vi "Get Event Selector Name QD.vi"(8 "error in (no error)":errorcluster, 10 "Library Ref in":refnum<vi>, 11 "VI Ref in":refnum<vi>) -> (0 "error out":errorcluster, 2 "Library Ref out":refnum<vi>, 3 "VI Ref out":refnum<vi>, 4 "Event Selector Name":string)   [LabVIEW 2017]
doc: "Returns the Event Selector name related to the selected SubVI."
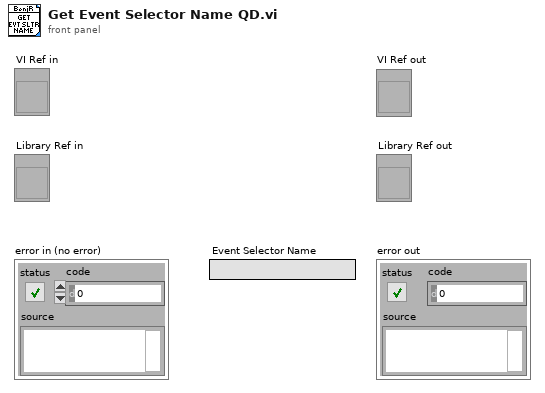
[diagram p1: front panel]
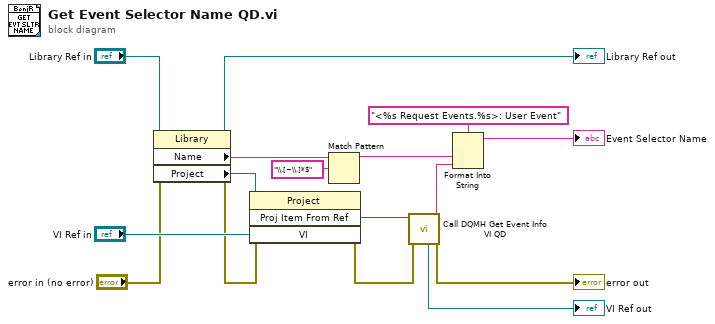
[diagram p0: block diagram]
diagram:
  n1 = property class="Library"(reference="Library Ref in", error in="error in (no error)") -> (reference out=→"Library Ref out":refnum<vi>, error out=w8:errorcluster, "Name"=w11:string, "Project"=w13:refnum<vi>)
  n2 = invoke class="Project" method="Proj Item From Ref"(reference=w13, error in=w8, "VI"="VI Ref in") -> (error out=w4:errorcluster, "ProjItemFromRef"=w5:refnum<vi>)  [unwired: 1 in, 2 out]
  n3 = Match Pattern(string=w11, regular expression="\\.[~\\.]*$") -> (before substring=w14:string)  [unwired: 4 out]
  n4 = call "Call DQMH Get Event Info VI QD.vi"("error in (no error)"=w4, "ProjectItem in"=w5) -> ("error out"=→"error out":errorcluster, "Event Name"=w1:string, "VI Ref"=→"VI Ref out":refnum<vi>)  [unwired: 7 in]
  n5 = Format Into String(format string="<%s Request Events.%s>: User Event" ("regular expression"), w14, w1) -> (resulting string=→"Event Selector Name":string)  [unwired: 2 in, 1 out]
